vi "Describe Call Comparison.vi"(11 "VI Call in":refnum<class "VI Call.lvclass">) -> (3 "delimited string":string)   [LabVIEW 2020, in "Any Inputs Comparator.lvclass"]
uses:
  Any Inputs Comparator.lvclass
  Core/VI Call/VI Call.lvclass
  Any Inputs Comparator.lvclass/Any Inputs Comparator.ctl
  Core/Comparator/Comparator.lvclass
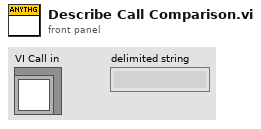
[diagram p1: front panel]
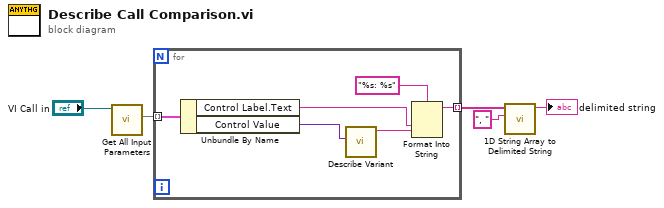
[diagram p0: block diagram]
diagram:
  n1 = call-dynamic "Get All Input Parameters.vi"("VI Call in"="VI Call in") -> ("Input Parameters"=w4:map{string, variant})  [unwired: 9 in, 1 out]
  n2 = for {
    tunnel: w4 -> [w11] mode=indexing
    tunnel: [w8] -> w1 mode=indexing
    n3 = Unbundle By Name(w11) -> ("Control Label.Text"=w9:string, "Control Value"=w7:variant)
    n4 = call "Describe Variant.vi"("Variant"=w7) -> ("Description with Type"=w6:string)  [unwired: 8 in, 2 out]
    n5 = Format Into String(format string="%s: %s", w9, w6) -> (resulting string=w8:string)  [unwired: 2 in, 1 out]
  }
  n6 = call <vilib>:"1D String Array to Delimited String.vi"("delimiter"=", ", "string array"=w1) -> ("delimited string"=→"delimited string":string)  [unwired: 9 in]
